vi "Telem Tool Get Device Data From Report.vi"() -> ()   [LabVIEW 2010]
panel:
  out "Number of Lines Processed":i32
  out "HV_CALS":string[](array[string])
  out "GEN_CALS":string[](array[string])
  out "CHAN_CALS":string[](array[string])
  out "STIM_TRIM":string[](array[string])
  out "TRIM_Z":string[](array[string])
  out "TRIM_P":string[](array[string])
  out "PULSE_CONST":string[](array[string])
  out "text":string
  out "PRGM_CONST":string[](array[string])
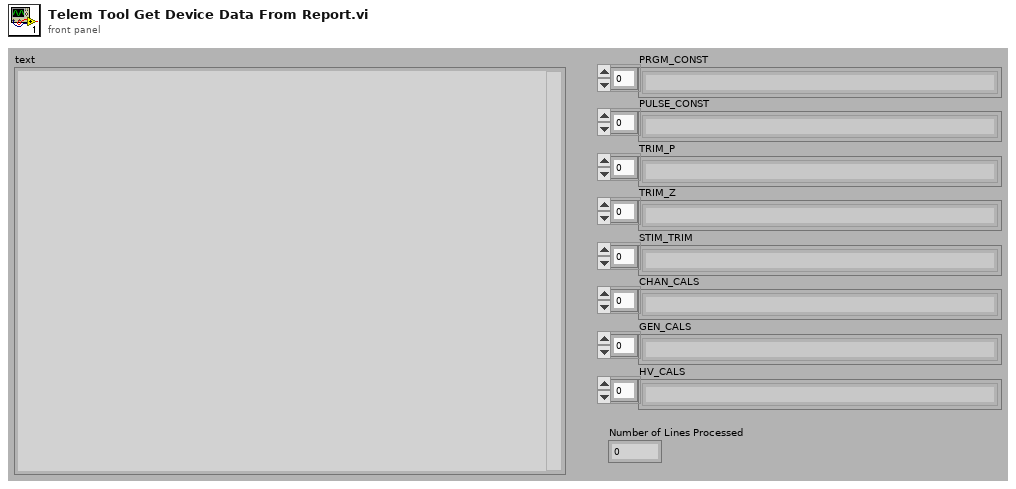
[diagram p1: front panel]
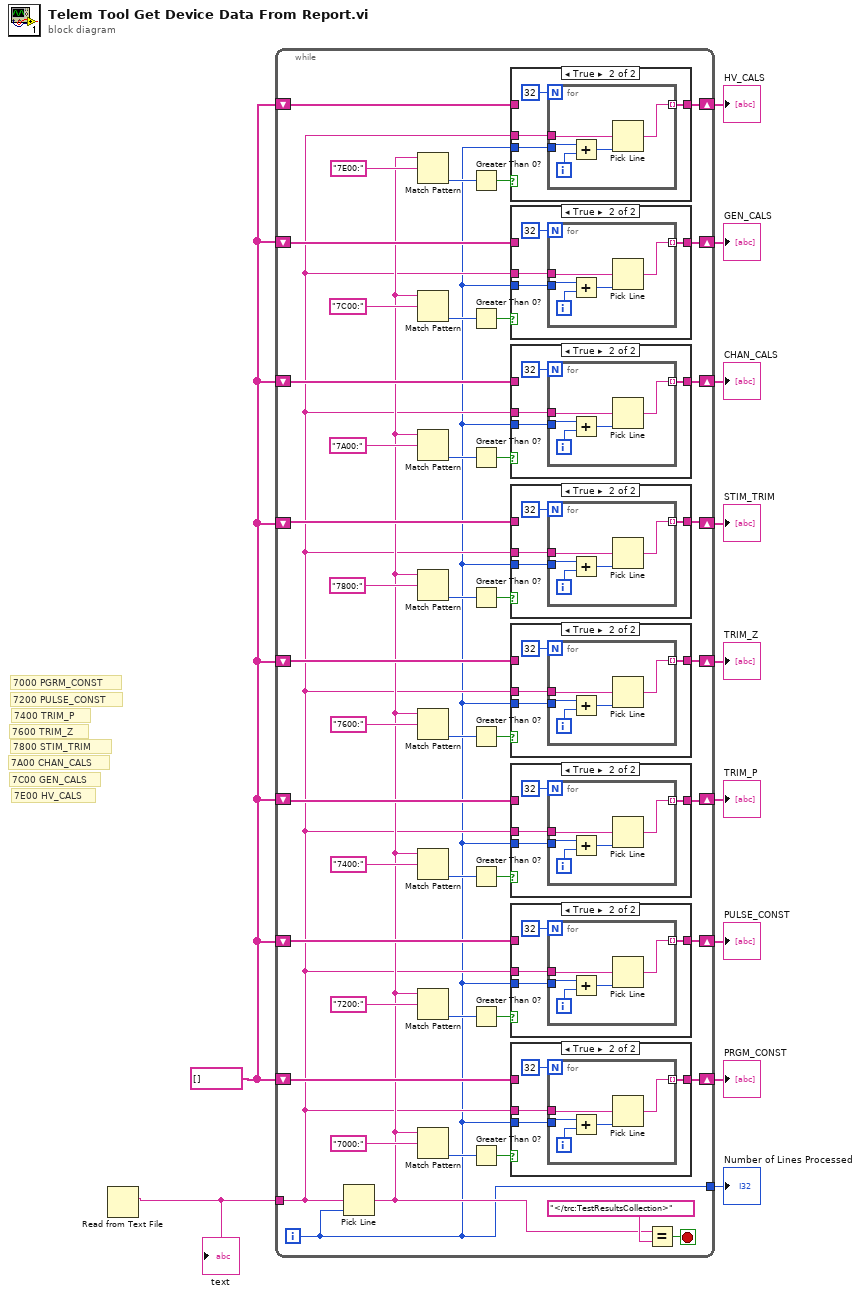
[diagram p0: block diagram]
diagram:
  w3 = string[] []
  # "7E00 HV_CALS"
  # "7C00 GEN_CALS"
  # "7A00 CHAN_CALS"
  # "7800 STIM_TRIM"
  # "7600 TRIM_Z"
  # "7400 TRIM_P"
  # "7200 PULSE_CONST"
  # "7000 PGRM_CONST"
  n1 = Read from Text File() -> (text=w11:string)  [unwired: 4 in, 3 out]
  "text" <- w11
  n2 = while {
    tunnel: w11 -> [w15]
    shift-right: [w53] -> w10
    shift-left: w3 -> [w52]
    shift-right: [w46] -> w9
    shift-left: w3 -> [w45]
    shift-right: [w41] -> w8
    shift-left: w3 -> [w40]
    shift-right: [w35] -> w7
    shift-left: w3 -> [w36]
    shift-right: [w31] -> w6
    shift-left: w3 -> [w30]
    shift-right: [w25] -> w5
    shift-left: w3 -> [w26]
    shift-right: [w21] -> w4
    shift-left: w3 -> [w20]
    shift-right: [w13] -> w2
    shift-left: w3 -> [w14]
    tunnel: [w12] -> w1
    i -> [w12]
    stop <- w50 stop-if-true
    n3 = Pick Line(multi-line string=w15, line index=w12) -> (output string=w16:string)  [unwired: 1 in]
    n4 = Match Pattern(string=w16, regular expression="7E00:") -> (offset past match=w18:i32)  [unwired: 1 in, 3 out]
    n5 = Match Pattern(string=w16, regular expression="7C00:") -> (offset past match=w23:i32)  [unwired: 1 in, 3 out]
    n6 = Match Pattern(string=w16, regular expression="7A00:") -> (offset past match=w28:i32)  [unwired: 1 in, 3 out]
    n7 = Match Pattern(string=w16, regular expression="7800:") -> (offset past match=w33:i32)  [unwired: 1 in, 3 out]
    n8 = Match Pattern(string=w16, regular expression="7600:") -> (offset past match=w38:i32)  [unwired: 1 in, 3 out]
    n9 = Match Pattern(string=w16, regular expression="7400:") -> (offset past match=w43:i32)  [unwired: 1 in, 3 out]
    n10 = Match Pattern(string=w16, regular expression="7200:") -> (offset past match=w48:i32)  [unwired: 1 in, 3 out]
    n11 = Match Pattern(string=w16, regular expression="7000:") -> (offset past match=w55:i32)  [unwired: 1 in, 3 out]
    n12 = Greater Than 0?(x=w18) -> (x > 0?=w17:bool)
    n13 = Greater Than 0?(x=w23) -> (x > 0?=w22:bool)
    n14 = Greater Than 0?(x=w28) -> (x > 0?=w27:bool)
    n15 = Greater Than 0?(x=w33) -> (x > 0?=w32:bool)
    n16 = Greater Than 0?(x=w38) -> (x > 0?=w37:bool)
    n17 = Greater Than 0?(x=w43) -> (x > 0?=w42:bool)
    n18 = Greater Than 0?(x=w48) -> (x > 0?=w47:bool)
    n19 = Greater Than 0?(x=w55) -> (x > 0?=w54:bool)
    n20 = case shown="True" w17 {
      tunnel: w15 -> [_ w61]
      tunnel: [w57 w59] -> w13
      tunnel: w14 -> [w57 _]
      tunnel: w12 -> [_ w58]
      frame False {
      }
      frame True {
        n21 = for {
          N: 32 -> [_]
          tunnel: w61 -> [w66]
          tunnel: [w65] -> w59 mode=indexing
          tunnel: w58 -> [w64]
          i -> [w63]
          n22 = Add(x=w64, y=w63) -> (x+y=w62:i32)
          n23 = Pick Line(multi-line string=w66, line index=w62) -> (output string=w65:string)  [unwired: 1 in]
        }
      }
    }
    n24 = case shown="True" w22 {
      tunnel: w15 -> [_ w71]
      tunnel: [w67 w69] -> w21
      tunnel: w20 -> [w67 _]
      tunnel: w12 -> [_ w68]
      frame False {
      }
      frame True {
        n25 = for {
          N: 32 -> [_]
          tunnel: w71 -> [w76]
          tunnel: [w75] -> w69 mode=indexing
          tunnel: w68 -> [w74]
          i -> [w73]
          n26 = Add(x=w74, y=w73) -> (x+y=w72:i32)
          n27 = Pick Line(multi-line string=w76, line index=w72) -> (output string=w75:string)  [unwired: 1 in]
        }
      }
    }
    n28 = case shown="True" w27 {
      tunnel: w15 -> [_ w81]
      tunnel: [w77 w79] -> w25
      tunnel: w26 -> [w77 _]
      tunnel: w12 -> [_ w78]
      frame False {
      }
      frame True {
        n29 = for {
          N: 32 -> [_]
          tunnel: w81 -> [w86]
          tunnel: [w85] -> w79 mode=indexing
          tunnel: w78 -> [w84]
          i -> [w83]
          n30 = Add(x=w84, y=w83) -> (x+y=w82:i32)
          n31 = Pick Line(multi-line string=w86, line index=w82) -> (output string=w85:string)  [unwired: 1 in]
        }
      }
    }
    n32 = case shown="True" w32 {
      tunnel: w15 -> [_ w91]
      tunnel: [w87 w89] -> w31
      tunnel: w30 -> [w87 _]
      tunnel: w12 -> [_ w88]
      frame False {
      }
      frame True {
        n33 = for {
          N: 32 -> [_]
          tunnel: w91 -> [w96]
          tunnel: [w95] -> w89 mode=indexing
          tunnel: w88 -> [w94]
          i -> [w93]
          n34 = Add(x=w94, y=w93) -> (x+y=w92:i32)
          n35 = Pick Line(multi-line string=w96, line index=w92) -> (output string=w95:string)  [unwired: 1 in]
        }
      }
    }
    n36 = case shown="True" w37 {
      tunnel: w15 -> [_ w101]
      tunnel: [w97 w99] -> w35
      tunnel: w36 -> [w97 _]
      tunnel: w12 -> [_ w98]
      frame False {
      }
      frame True {
        n37 = for {
          N: 32 -> [_]
          tunnel: w101 -> [w106]
          tunnel: [w105] -> w99 mode=indexing
          tunnel: w98 -> [w104]
          i -> [w103]
          n38 = Add(x=w104, y=w103) -> (x+y=w102:i32)
          n39 = Pick Line(multi-line string=w106, line index=w102) -> (output string=w105:string)  [unwired: 1 in]
        }
      }
    }
    n40 = case shown="True" w42 {
      tunnel: w15 -> [_ w111]
      tunnel: [w107 w109] -> w41
      tunnel: w40 -> [w107 _]
      tunnel: w12 -> [_ w108]
      frame False {
      }
      frame True {
        n41 = for {
          N: 32 -> [_]
          tunnel: w111 -> [w116]
          tunnel: [w115] -> w109 mode=indexing
          tunnel: w108 -> [w114]
          i -> [w113]
          n42 = Add(x=w114, y=w113) -> (x+y=w112:i32)
          n43 = Pick Line(multi-line string=w116, line index=w112) -> (output string=w115:string)  [unwired: 1 in]
        }
      }
    }
    n44 = case shown="True" w47 {
      tunnel: w15 -> [_ w121]
      tunnel: [w117 w119] -> w46
      tunnel: w45 -> [w117 _]
      tunnel: w12 -> [_ w118]
      frame False {
      }
      frame True {
        n45 = for {
          N: 32 -> [_]
          tunnel: w121 -> [w126]
          tunnel: [w125] -> w119 mode=indexing
          tunnel: w118 -> [w124]
          i -> [w123]
          n46 = Add(x=w124, y=w123) -> (x+y=w122:i32)
          n47 = Pick Line(multi-line string=w126, line index=w122) -> (output string=w125:string)  [unwired: 1 in]
        }
      }
    }
    n48 = case shown="True" w54 {
      tunnel: w15 -> [_ w131]
      tunnel: [w127 w129] -> w53
      tunnel: w52 -> [w127 _]
      tunnel: w12 -> [_ w128]
      frame False {
      }
      frame True {
        n49 = for {
          N: 32 -> [_]
          tunnel: w131 -> [w136]
          tunnel: [w135] -> w129 mode=indexing
          tunnel: w128 -> [w134]
          i -> [w133]
          n50 = Add(x=w134, y=w133) -> (x+y=w132:i32)
          n51 = Pick Line(multi-line string=w136, line index=w132) -> (output string=w135:string)  [unwired: 1 in]
        }
      }
    }
    n52 = Equal?(x=w16, y="</trc:TestResultsCollection>") -> (x = y?=w50:bool)
  }
  "PRGM_CONST" <- w10
  "PULSE_CONST" <- w9
  "TRIM_P" <- w8
  "TRIM_Z" <- w7
  "STIM_TRIM" <- w6
  "CHAN_CALS" <- w5
  "GEN_CALS" <- w4
  "HV_CALS" <- w2
  "Number of Lines Processed" <- w1
